vi "CurrentDate.vi"() -> (3 "当前日期时间":string)   [LabVIEW 2015]
panel:
  # "Date are in the following format YYYY-MM-DD HH:MM:SS ±HHMM \nFor example “2001-03-24 10:45:32 +0600”"
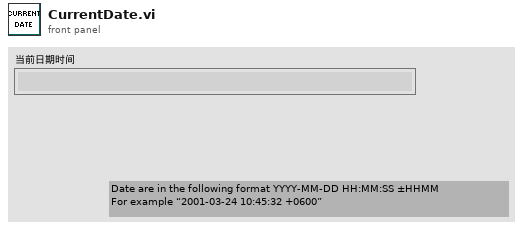
[diagram p1: front panel]
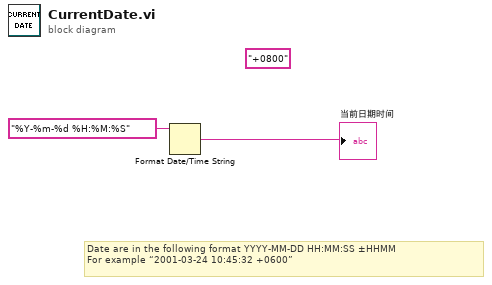
[diagram p0: block diagram]
diagram:
  (unwired) "+0800" ("字符串")
  # "Date are in the following format YYYY-MM-DD HH:MM:SS ±HHMM \nFor example “2001-03-24 10:45:32 +0600”"
  n1 = Format Date/Time String(time format string (%c)="%Y-%m-%d %H:%M:%S" ("时间格式字符串(%c)")) -> (date/time string=→"当前日期时间":string)  [unwired: 2 in]
